vi "ComputeRelativeZJoystickPosition.vi"(5 "Joystick Axis Info":T1, 6 "Joystick Offset":T2, 7 "reference":refnum<vi>) -> (3 "Rel Z Pos":T3)   [LabVIEW 2014]
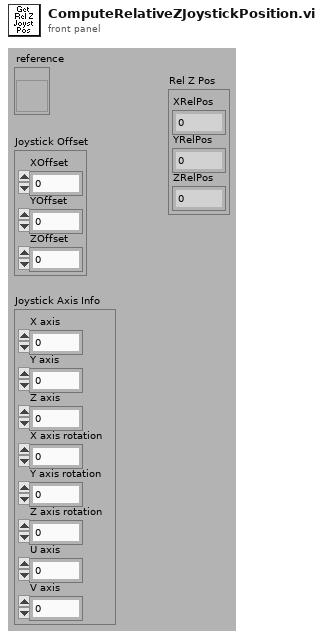
[diagram p1: front panel]
types:
  T1 = cluster{"X axis":i32, "Y axis":i32, "Z axis":i32, "X axis rotation":i32, "Y axis rotation":i32, "Z axis rotation":i32, "U axis":i32, "V axis":i32}
  T2 = cluster{"XOffset":i32, "YOffset":i32, "ZOffset":i32}
  T3 = cluster{"XRelPos":i32, "YRelPos":i32, "ZRelPos":i32}
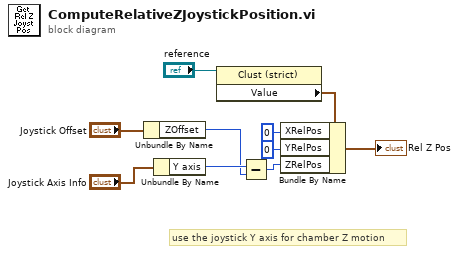
[diagram p0: block diagram]
diagram:
  # "use the joystick Y axis for chamber Z motion"
  n1 = Unbundle By Name("Joystick Offset") -> ("ZOffset"=w1:i32)
  n2 = Unbundle By Name("Joystick Axis Info") -> ("Y axis"=w2:i32)
  n3 = property class="Clust (strict)"(reference="reference") -> ("Value"=w9:T3)  [unwired: 1 in, 2 out]
  n4 = Subtract(x=w2, y=w1) -> (x-y=w5:i32)
  n5 = Bundle By Name(cluster=w9, "XRelPos"=0, "YRelPos"=0, "ZRelPos"=w5) -> (→"Rel Z Pos":T3)
